vi "Finite Sample Start.vi"(7 "Number of Samples":u16, 8 "Error In":errorcluster, 9 "Acquition Speed (HZ)":u16, 10 "Analog Input Pin":u8, 11 "ChipKit Resource":T1={"COM Port"="", "Board Type"=enum."ChipKit uC32", "Connection Type"=enum."USB / Serial", "Baud Rate (115200)"=15, "Bytes Per Packet (15)"=15}) -> (0 "Error Out":errorcluster, 3 "ChipKit Resource":T1={"COM Port"="", "Board Type"=enum."ChipKit uC32", "Connection Type"=enum."USB / Serial", "Baud Rate (115200)"=15, "Bytes Per Packet (15)"=15})   [LabVIEW 2011, in "LabVIEW Interface for ChipKit.lvlib"]
doc: "This VI configures and starts a finite execution on the Arduino. After this VI is run the arduino will start to output data to the serial port continuously until the number of samples set is reached."
uses:
  LabVIEW Interface for ChipKit.lvlib
  Private/Type Defs/Chipkit Resource.ctl
  Private/Type Defs/Board Type.ctl
  Private/Type Defs/Connection Type.ctl
  Private/Type Defs/Command.ctl
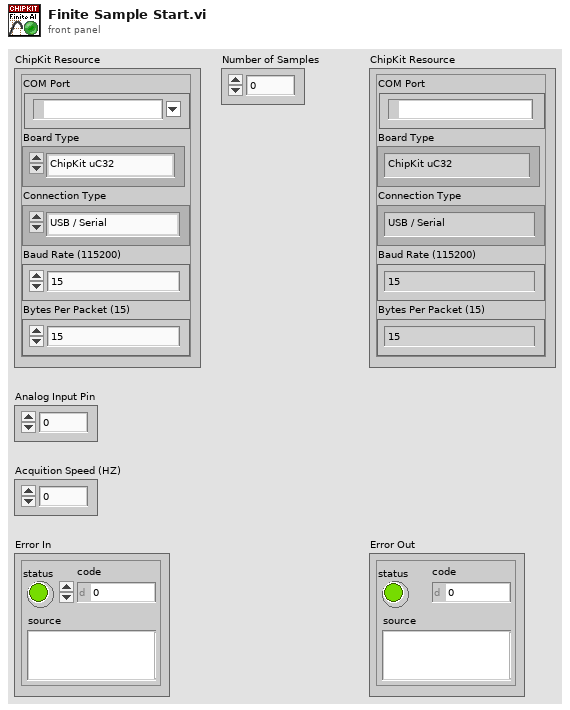
[diagram p1: front panel]
types:
  T1 = typedef "LabVIEW Interface for ChipKit.lvlib/Chipkit Resource.ctl" = cluster{"COM Port":refnum<visa-resource-name>, "Board Type":T2, "Connection Type":T3, "Baud Rate (115200)":u32, "Bytes Per Packet (15)":u32}
  T2 = typedef "LabVIEW Interface for ChipKit.lvlib/Board Type.ctl" = enum16{"ChipKit uC32", "ChipKit Uno32", "ChipKit Max32"}
  T3 = typedef "LabVIEW Interface for ChipKit.lvlib/Connection Type.ctl" = enum8{"USB / Serial", "XBEE", "BlueSmirf (Bluetooth)"}
  T4 = typedef "LabVIEW Interface for ChipKit.lvlib/Command.ctl" = enum8{"setArduinoMode", "flushSerial", "setPinMode", "digitalWritePin", "digitalWritePort", "tone", "digitalReadPin", "digitalReadPort", "analogReadPin", "analogReadPort", "pwmWritePin", "pwmWritePort", "sevenSegment_Configure", "sevenSegment_Write", "I2C Init", "I2C Write", "I2C Read", "SPI Init", "SPI Set Bit Order", "SPI Set Clock Divider", "SPI Set Data Mode", "SPI Send / Receive", "SPI Close", "Servo Set Num Servos", "Servo Config Servo", "Servo Write Angle", "Servo Read Angle", "Servo Write Pulse Width", "Servo Read Pulse Width", "Servo Detach", "LCD Init", "LCD Set Size", "LCD Set Cursor Mode", "LCD Clear", "LCD Set Cursor Position", "LCD Print", "LCD Display Power", "LCD Scroll Display", "LCD Autoscroll", "LCD Print Direction", "LCD Create Custom Char", "LCD Print Custom Char", "contAcqOn", "contAcqOff", "getFirmwareVersion", "FiniteSampleStart", "NA", "NA2", "Conifg Stepper", "Stepper Write", "Stepper Detach", "Stepper Steps To Go", "Config DO Port", "Config DI Port", "UART2 Open", "UART2 Write", "UART2 Bytes Available", "UART2 Read"}
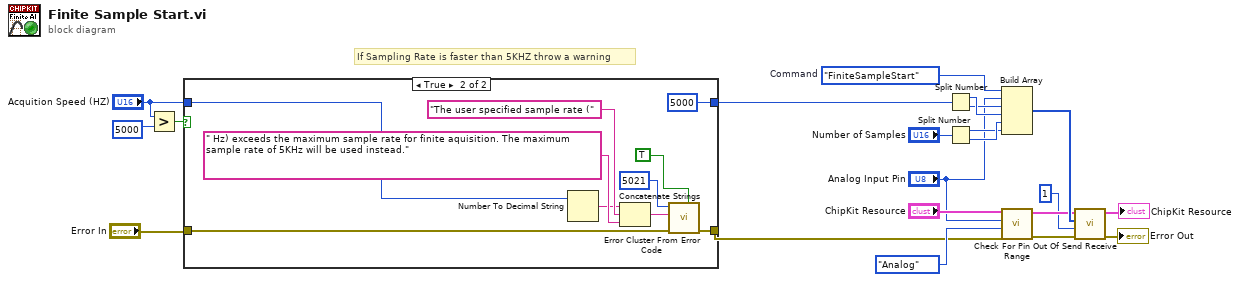
[diagram p0: block diagram]
diagram:
  w20 = Command."FiniteSampleStart"  # Command
  # "If Sampling Rate is faster than 5KHZ throw a warning"
  n1 = Greater?(x="Acquition Speed (HZ)", y=u16 5000) -> (0:w6:bool)
  n2 = case shown="True" w6 {
    tunnel: [w23 w28] -> w3
    tunnel: "Error In" -> [w23 w27]
    tunnel: "Acquition Speed (HZ)" -> [w22 w26]
    tunnel: [w22 u32 5000 ("Acquition Speed")] -> w2
    frame False {
    }
    frame True {
      n3 = Number To Decimal String(number=w26) -> (decimal integer string=w30:string)  [unwired: 1 in]
      n4 = Concatenate Strings(w30, "The user specified sample rate (", " Hz) exceeds the maximum sample rate for finite aquisition. The maximum sample rate of 5KHz will be used instead." ("source")) -> (w25:string)
      n5 = call <vilib>:"Error Cluster From Error Code.vi"("is warning? (False)"=TRUE, "error in (no error)"=w27, "error message (\"\")"=w25, "error code (0)"=5021) -> ("error out"=w28:errorcluster)  [unwired: 5 in]
    }
  }
  n6 = Split Number(x=w2) -> (hi(x)=w19:u16, lo(x)=w18:u16)
  n7 = Split Number(x="Number of Samples") -> (hi(x)=w15:u8, lo(x)=w16:u8)
  n8 = Build Array(w20, "Analog Input Pin", w18, w19, w16, w15) -> (w14:u16[])
  n9 = call "Check For Pin Out Of Range.vi"("Error In"=w3, "Pin Type"=enum16{"Analog", "Digital"}."Analog", "User Pin Number"="Analog Input Pin", "Arduino Resource"="ChipKit Resource") -> ("Error Out"=w13:errorcluster, "Arduino Resource"=w11:T1)  [unwired: 6 in]
  n10 = call "Send Receive.vi"("Error In"=w13, "Bytes To Read (0)"=u8 1, "Data"=w14, "ChipKit Resource"=w11) -> ("Error Out"=→"Error Out":errorcluster, "ChipKit Resource"=→"ChipKit Resource":T1)  [unwired: 5 in, 1 out]
